vi "Angle to Tape.vi"(9 "Distance To Target (ft)":dbl, 10 "Y":dbl, 11 "X":dbl) -> (1 "Distance to Wall (ft)":dbl, 2 "Polar Plot":picture, 3 "Angle from Robot (deg)":dbl)   [LabVIEW 2013]
uses:
  <vilib>/Utility/miscctls.llb/LVBoundsTypeDef.ctl
panel:
  in  "Plot Color":u32(colorbox)=16715776
  in  "Grid Color":u32(colorbox)
  in  "Visible Section":u16(ring)=4
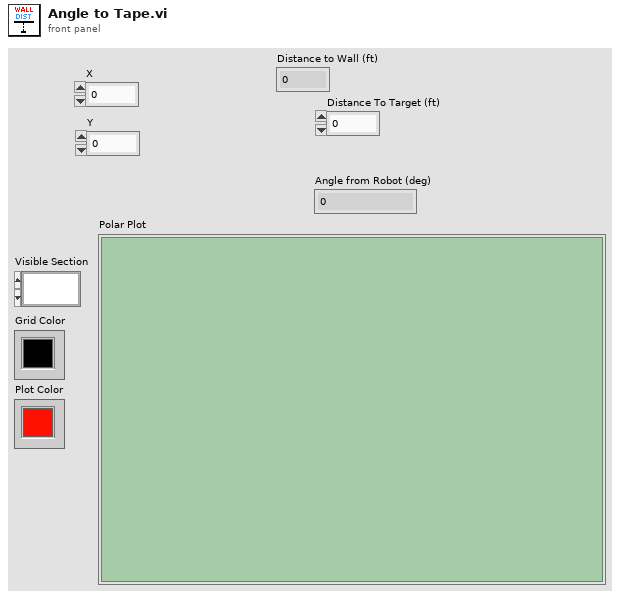
[diagram p1: front panel]
types:
  T1 = typedef "LVBoundsTypeDef.ctl" = cluster{"Width":u32, "Height":u32}
  T2 = cluster{"maximum":dbl, "minimum":dbl, "clip to min":bool, "log?(F)":bool, "grid color":u32, "plot color":u32, "format and precision":cluster{"format":enum8{"Decimal", "Scientific", "Engineering", "Binary", "Octal", "Hex"}, "precision":u8}, "visible section":u16}
  T3 = cluster{"Distance To Target (ft)":dbl, "Radius":dbl}[]
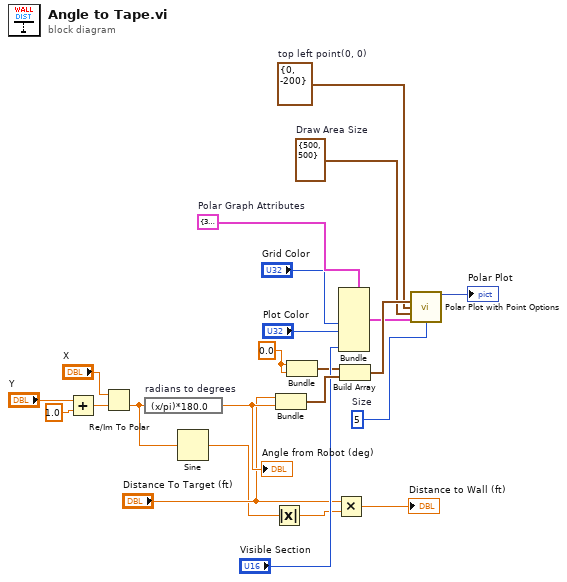
[diagram p0: block diagram]
diagram:
  w6 = T1 {"Width"=500, "Height"=500}  # Draw Area Size
  w7 = cluster{"x":i16, "y":i16} {"x"=0, "y"=-200}  # top left point(0, 0)
  w13 = u16 5  # Size
  w14 = 0.0 ("Radius")
  w19 = T2 {"maximum"=30.0, "minimum"=0.0, "clip to min"=FALSE, "log?(F)"=FALSE, "grid color"=6710886, "plot color"=65280, "format and precision"={"format"=enum."Decimal", "precision"=1}, "visible section"=0}  # Polar Graph Attributes
  n1 = Add(x="Y", y=1.0) -> (x+y=w11:dbl)
  n2 = Re/Im To Polar(2:w11, 3:"X") -> (0:w3:dbl)  [unwired: 1 out]
  n3 = expression code="(x/pi)*180.0" "radians to degrees"(w3) -> (w22:dbl)
  "Angle from Robot (deg)" <- w22
  n4 = Sine(x=w3) -> (sin(x)=w2:dbl)
  n5 = Absolute Value(x=w2) -> (abs(x)=w1:dbl)
  n6 = Bundle("Distance To Target (ft)"="Distance To Target (ft)", w22) -> (w21:cluster{"Distance To Target (ft)":dbl, dbl})  [unwired: 1 in]
  n7 = Bundle("Radius"=w14, "Radius"=w14) -> (w15:cluster{"Radius":dbl, "Radius":dbl})  [unwired: 1 in]
  n8 = Multiply(x="Distance To Target (ft)", y=w1) -> (x*y=→"Distance to Wall (ft)":dbl)
  n9 = Bundle(cluster=w19, "grid color"="Grid Color", "plot color"="Plot Color", "visible section"="Visible Section") -> (w8:T2)  [unwired: 5 in]
  n10 = Build Array(w15, w21) -> (w20:T3)
  n11 = call <vilib>:"Polar Plot with Point Options.vi"("data array [mag, phase (deg)]"=w20, "top left point(0, 0)"=w7, "dimensions (w,h)"=w6, "polar attributes"=w8, "Size"=w13) -> ("new picture"=→"Polar Plot":picture)  [unwired: 10 in]
